vi "Client Read Configuration.vi"(11 "configuration file path":path=path "c:/clientconfig.ini") -> (0 "error out":errorcluster, 2 "valid data":bool, 3 "Host IP Address":string)   [LabVIEW 2013]
uses:
  <vilib>/Utility/config.llb/Read Key (String).vi
  Client Configuration.vi
  <vilib>/Utility/config.llb/NI_LVConfig.lvlib
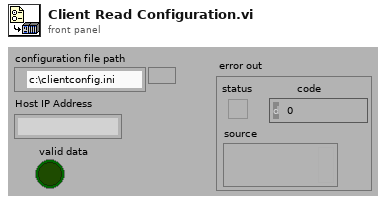
[diagram p1: front panel]
types:
  T1 = typedef "NI_LVConfig.lvlib/Config Data RefNum.ctl" = refnum<k1>
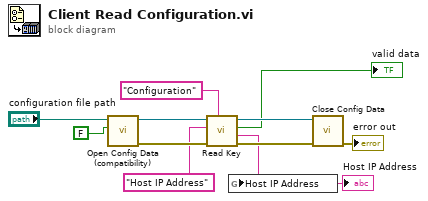
[diagram p0: block diagram]
diagram:
  n1 = call <vilib>:"Open Config Data (compatibility).vi"("create file if necessary (T)"=FALSE ("create file if necessary? (T)"), "configuration file path"="configuration file path") -> ("error out"=w10:errorcluster, "refnum"=w9:T1)  [unwired: 7 in, 1 out]
  n2 = call-poly <vilib>:"Read Key.vi"("section"="Configuration", "error in (no error)"=w10, "key"="Host IP Address", "refnum"=w9) -> ("error out"=w8:errorcluster, "value"=w4:string, "found?"=→"valid data":bool, "refnum out"=w7:T1)  [unwired: 4 in]
  "Host IP Address" <- w4
  n3 = global write "Client Configuration.vi" "Host IP Address"(w4) -> ()
  n4 = call <vilib>:"Close Config Data.vi"("error in (no error)"=w8, "refnum"=w7) -> ("error out"=→"error out":errorcluster)  [unwired: 8 in, 1 out]
